vi "Lights.vi"(10 "Colour":T1(ring)=enum."Blue") -> ()   [LabVIEW 2019]
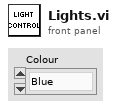
[diagram p1: front panel]
types:
  T1 = enum16{"Blue + Yellow", "Green", "Hot Pink", "Yellow", "Blue", "Red"}
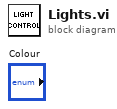
[diagram p0: block diagram]
diagram:
